vi "toISS-Epoch.vi"(11 "Epoch in":refnum<class "Epoch.lvclass">) -> (2 "ISS Time":fxp<+,40,40>, 3 "Epoch":refnum<class "Epoch.lvclass">)   [LabVIEW 2013, in "Epoch.lvclass"]
uses:
  Epoch.lvclass
  Epoch.lvclass/Epoch.ctl
panel:
  out "x*y":u8
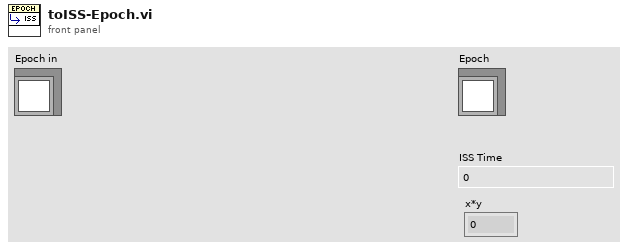
[diagram p1: front panel]
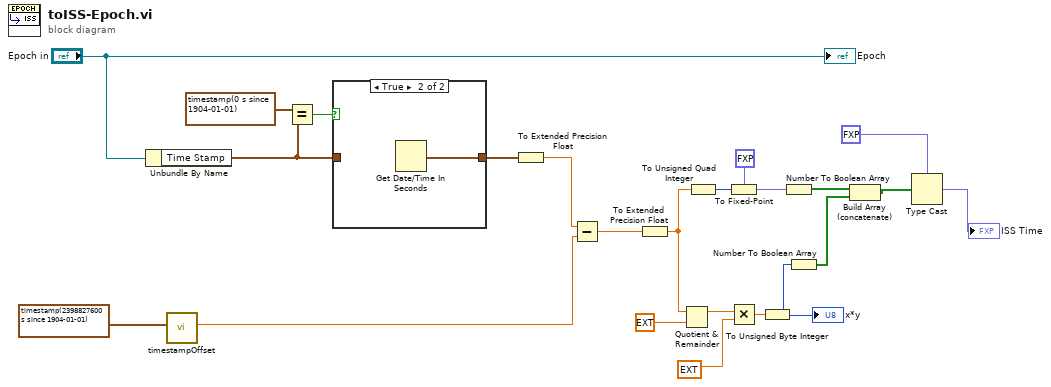
[diagram p0: block diagram]
diagram:
  n1 = Unbundle By Name("Epoch in") -> ("Time Stamp"=w15:timestamp)
  n2 = call "timestampOffset.vi"("Reference Time"=timestamp(2398827600 s since 1904-01-01) ("Timestamp")) -> ("Timestamp Offset"=w19:ext)  [unwired: 10 in]
  n3 = Equal?(x=timestamp(0 s since 1904-01-01), y=w15) -> (x = y?=w17:bool)
  n4 = case shown="True" w17 {
    tunnel: [w24 w25] -> w16
    tunnel: w15 -> [w24 _]
    frame False {
    }
    frame True {
      n5 = Get Date/Time In Seconds() -> (seconds since 1Jan1904=w25:timestamp)
    }
  }
  n6 = To Extended Precision Float(1:w16) -> (0:w21:ext)
  n7 = Subtract(x=w21, y=w19) -> (x-y=w22:ext)
  n8 = To Extended Precision Float(1:w22) -> (0:w8:ext)
  n9 = Quotient & Remainder(x=w8, y=ext 1.0) -> (x-y*floor(x/y)=w13:ext)  [unwired: 1 out]
  n10 = To Unsigned Quad Integer(1:w8) -> (0:w10:u64)
  n11 = To Fixed-Point(fixed-point type=fxp<+,32,32> 0.0 ("TReK GPS Epoch Time"), number=w10) -> (fixed-point=w7:fxp<+,32,32>)
  n12 = Multiply(x=w13, y=ext 255.0) -> (x*y=w11:ext)
  n13 = To Unsigned Byte Integer(number=w11) -> (unsigned 8bit integer=w6:u8)
  "x*y" <- w6
  n14 = Number To Boolean Array(number=w7) -> (Boolean array=w5:bool[])
  n15 = Number To Boolean Array(number=w6) -> (Boolean array=w4:bool[])
  n16 = Build Array (concatenate)(w5, w4) -> (w3:bool[])
  n17 = Type Cast(type=fxp<+,40,40> 0.0 ("TReK GPS Epoch Time"), x=w3) -> (*(type *) &x=→"ISS Time":fxp<+,40,40>)
  "Epoch" <- "Epoch in"
